vi "hw8p7_hickey.vi"() -> ()   [LabVIEW 2014]
uses:
  <vilib>/imath/engines/lvmath2/RunTimeEngine/Managers/WorkSpace/UID Generator.vi
  <vilib>/imath/engines/lvmath2/RunTimeEngine/RunTimeType/NIMS_RunTimeType_From StrictType (excl LVString).vi
  <instcachedir>/0/NIMS_RunTimeType_From StrictType (excl LVString)_15A5391EEA9C4AACB9955AC755B83D29.lvgen/NIMS_RunTimeType_From StrictType (excl LVString)_15A5391EEA9C4AACB9955AC755B83D29_000.vi
  <vilib>/imath/engines/lvmath2/RunTimeEngine/LocalVariableDefStatement/MC_LocalVariableDefStatement_Display.vi
  <vilib>/imath/engines/lvmath2/RunTimeEngine/Managers/SymbolTable/Clear UID.vi
  <vilib>/imath/engines/lvmath2/RunTimeEngine/NodeEndStatement/NIMS_NodeEndStatement_Output.vi
  <instcachedir>/0/NIMS_NodeEndStatement_Output_53EC0D466D134D7ABD903AC30B43404B.lvgen/NIMS_NodeEndStatement_Output_53EC0D466D134D7ABD903AC30B43404B_005.vi
  <vilib>/imath/engines/lvmath2/RunTimeEngine/ErrorHandling/NIMS_Finalize Error.vi
  <vilib>/imath/engines/lvmath2/RunTimeEngine/Managers/SymbolTable/NIMS_WorkSpace.lvlib
panel:
  out "XY Graph":cluster{dbl[], "x":dbl[]}(graph)
  in  "Numeric":i32
  # "330 is the number of iterations you need to be off \nby 5% (.1)"
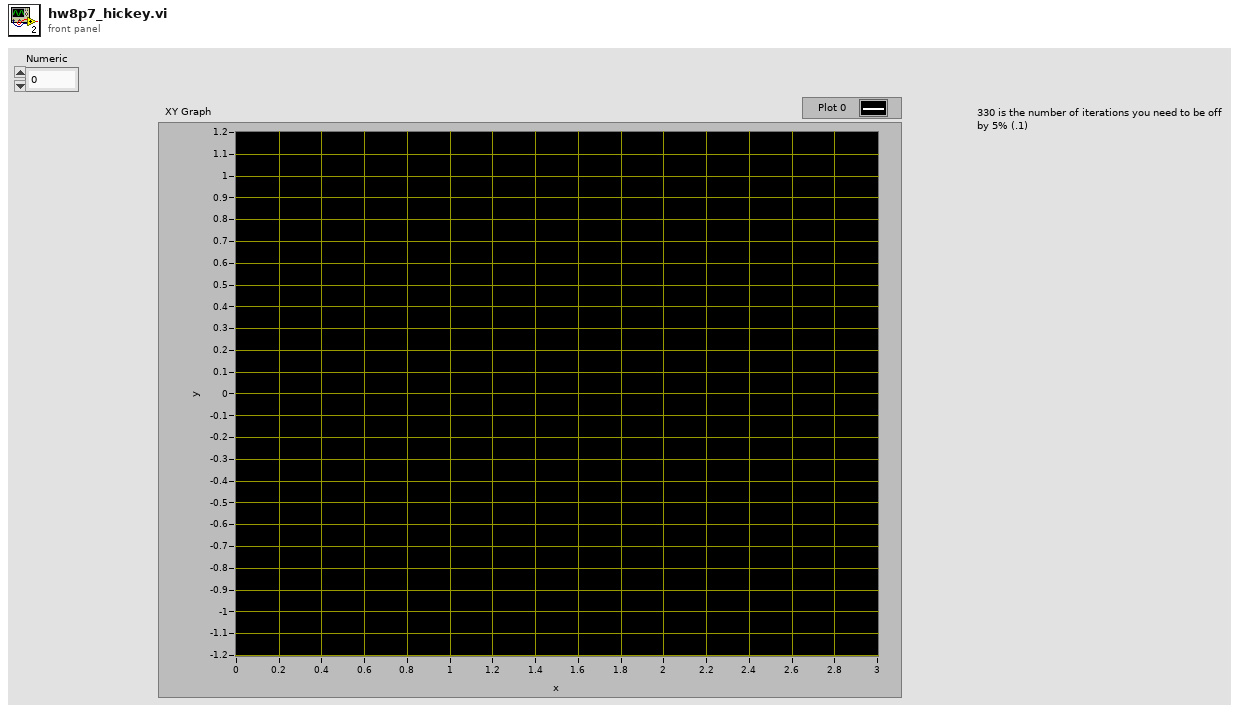
[diagram p1: front panel]
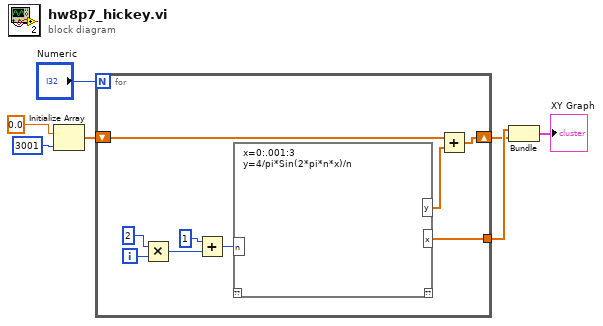
[diagram p0: block diagram]
diagram:
  n1 = Initialize Array(0.0 ("element"), 3001) -> (w5:dbl[])
  n2 = for {
    N: "Numeric" -> [_]
    shift-right: [w12] -> w1
    shift-left: w5 -> [w11]
    tunnel: [w8] -> w2
    i -> [w16]
    n3 = Multiply(x=2, y=w16) -> (x*y=w14:i32)
    n4 = Add(x=1, y=w14) -> (x+y=w10:i32)
    n5 = mathscript code="x=0:.001:3\ny=4/pi*Sin(2*pi*n*x)/n"("n"=w10) -> ("y"=w9:dbl[], "x"=w8:dbl[])  [unwired: 1 in, 1 out]
    n6 = Add(x=w11, y=w9) -> (x+y=w12:dbl[])
  }
  n7 = Bundle("x"=w2, w1) -> (→"XY Graph":cluster{"x":dbl[], dbl[]})  [unwired: 1 in]
